vi "Write Top_Left_Right_Bottom arrays.vi"(8 "error in (no error)":errorcluster, 10 "Top/Left/Right/Bottom arrays":T1 {"Position Integer" items=["Top", "Left", "Center", "Right", "Bottom"]}, 11 "PentaPanesGUI in":refnum<class "PentaPanes.lvclass">) -> (0 "error out":errorcluster, 3 "PentaPanesGUI out":refnum<class "PentaPanes.lvclass">)   [LabVIEW 2022 SP3, in "PentaPanesLibrary.lvlib" / "PentaPanes.lvclass"]
uses:
  PentaPanes.lvclass
  TopLeftRightBottomArrays.ctl
  PanePosition.ctl
  PentaPanes.lvclass/PentaPanes.ctl
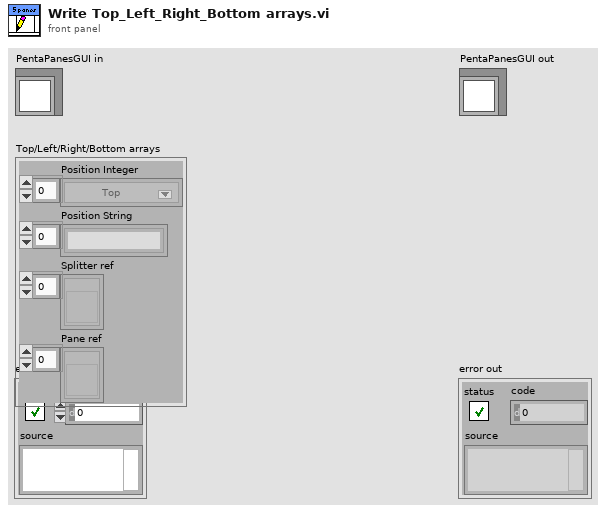
[diagram p1: front panel]
types:
  T1 = typedef "PentaPanesLibrary.lvlib/PentaPanes.lvclass/TopLeftRightBottomArrays.ctl" = cluster{"Position Integer":T2[], "Position String":string[], "Splitter ref":refnum<vi>[], "Pane ref":refnum<vi>[]}
  T2 = typedef "PentaPanesLibrary.lvlib/PentaPanes.lvclass/PanePosition.ctl" = u16
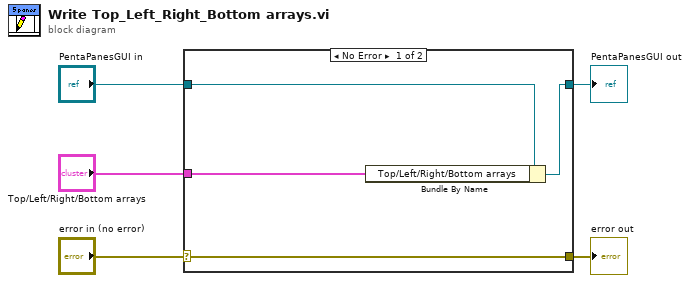
[diagram p0: block diagram]
diagram:
  n1 = case shown="No Error" "error in (no error)" {
    selector: "error in (no error)" -> [w9 w10]
    tunnel: [w9 w10] -> w4
    tunnel: [w7 w11] -> w2
    tunnel: "PentaPanesGUI in" -> [w8 w11]
    tunnel: "Top/Left/Right/Bottom arrays" -> [w6 _]
    frame No Error {
      n2 = Bundle By Name(cluster=w8, "Top/Left/Right/Bottom arrays"=w6) -> (w7:refnum<class "PentaPanes.lvclass">)
    }
    frame Error {
    }
  }
  "error out" <- w4
  "PentaPanesGUI out" <- w2
